vi "Profile_Max.vi"() -> (0 "New Values In":string[][](array[string])=[["Test data5"]], 1 "New Chs In":string[](array[string])=["30-10-03:New:Channel new5"])   [LabVIEW 2021]
uses:
  Results_plotter_Global.vi
  Data plotting/subVIs/Plot_Values_Global.vi
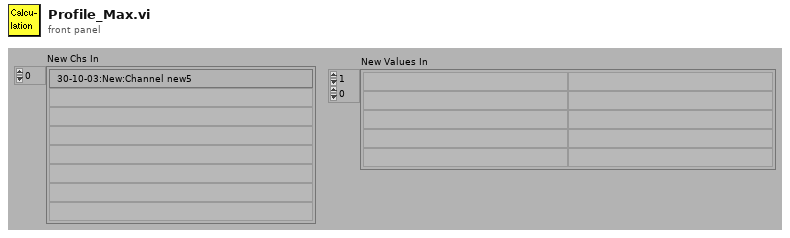
[diagram p1: front panel]
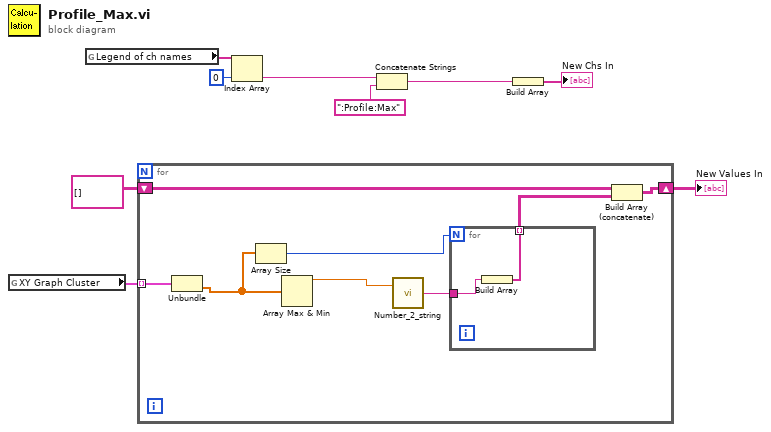
[diagram p0: block diagram]
diagram:
  n1 = global read "Plot_Values_Global.vi" "XY Graph Cluster"() -> (w1:cluster{dbl[], dbl[]}[])
  n2 = global read "Results_plotter_Global.vi" "Legend of ch names"() -> (w7:string[])
  n3 = for {
    tunnel: w1 -> [w17] mode=indexing
    shift-right: [w15] -> w5
    shift-left: string[][] [] -> [w16]
    n4 = Unbundle(w17) -> (w13:dbl[])  [unwired: 1 out]
    n5 = Array Size(array=w13) -> (size(s)=w11:i32)
    n6 = Array Max & Min(array=w13) -> (max value=w14:dbl)  [unwired: 3 out]
    n7 = call "Number_2_string.vi"("number"=w14) -> ("String"=w12:string)  [unwired: 1 in]
    n8 = for {
      N: w11 -> [_]
      tunnel: w12 -> [w19]
      tunnel: [w18] -> w10 mode=indexing
      n9 = Build Array(w19) -> (w18:string[])
    }
    n10 = Build Array (concatenate)(w16, w10) -> (w15:string[][])
  }
  "New Values In" <- w5
  n11 = Index Array(array=w7, index=0) -> (element=w3:string)
  n12 = Concatenate Strings(w3, ":Profile:Max" ("string")) -> (w2:string)
  n13 = Build Array(w2) -> (→"New Chs In":string[])
